vi "Amplitude and period panel.vi"() -> ()   [LabVIEW 2017]
uses:
  <vilib>/Analysis/6fits.llb/Remove Outliers (Index).vi
  control panel globals.vi
  <vilib>/Analysis/NI_AALPro.lvlib
  <vilib>/Analysis/NI_AALBase.lvlib
panel:
  in  "full x-range?":bool
  out "XY Graph":cluster{i32[], i16[]}[](graph)
  in  "discard outliers?":bool
  out "min T":dbl
  out "max T":dbl
  out "range (ms)":dbl format="%#_3f"
  out "average period (s)":dbl format="%.4f"
  out "stdev of period (ms)":dbl format="%_3f"
  out "L (m)":dbl
  in  "take snapshot":bool
  out "amplitude (mm)":sgl
  in  "clear orbit data":bool
  out "axis vs time":cluster{dbl[], dbl[]}(graph)
  out "deltaT vs. ampltidue":cluster{dbl[], dbl[]}[](graph)
  out "error out":errorcluster
  in  "log-log ?":bool
  in  "show most recent ____ seconds":dbl=5000.0
  out "period  vs time":cluster{dbl[], "dX/dt":dbl[]}(graph)
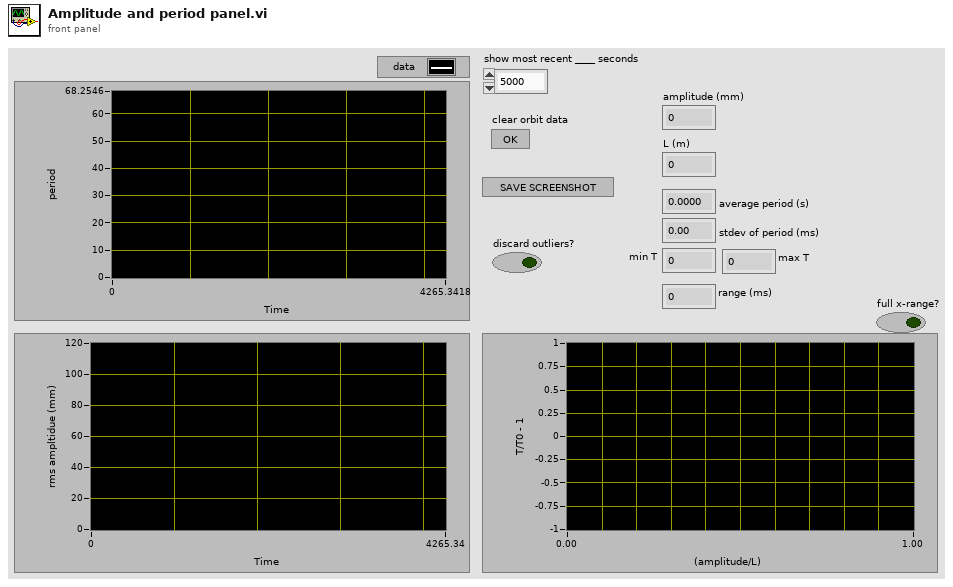
[diagram p1: front panel]
types:
  T1 = typedef "queue cluster.ctl" = cluster{"voltage":T2, "coil":T2, "mag":refnum<queue>, "accel":T2, "crossing":T2, "orbit fit":refnum<queue>, "pulse":T2, "mag0":T2, "fitLocation":refnum<queue>}
  T2 = typedef "reading queue.ctl" = refnum<queue>
  T3 = typedef "orbit parameters with crossing info.ctl" = cluster{"a":dbl, "b":dbl, "theta_axis":dbl, "dPhi":dbl, "BrV":dbl, "bob tilt":dbl, "phi0":dbl, "phi_dot":dbl, "x0":dbl, "y0":dbl, "z0":dbl, "mid crossing time":dbl, "most recent crossing number":dbl, "most recent crossing slope":dbl, "most recent crossing period":dbl}
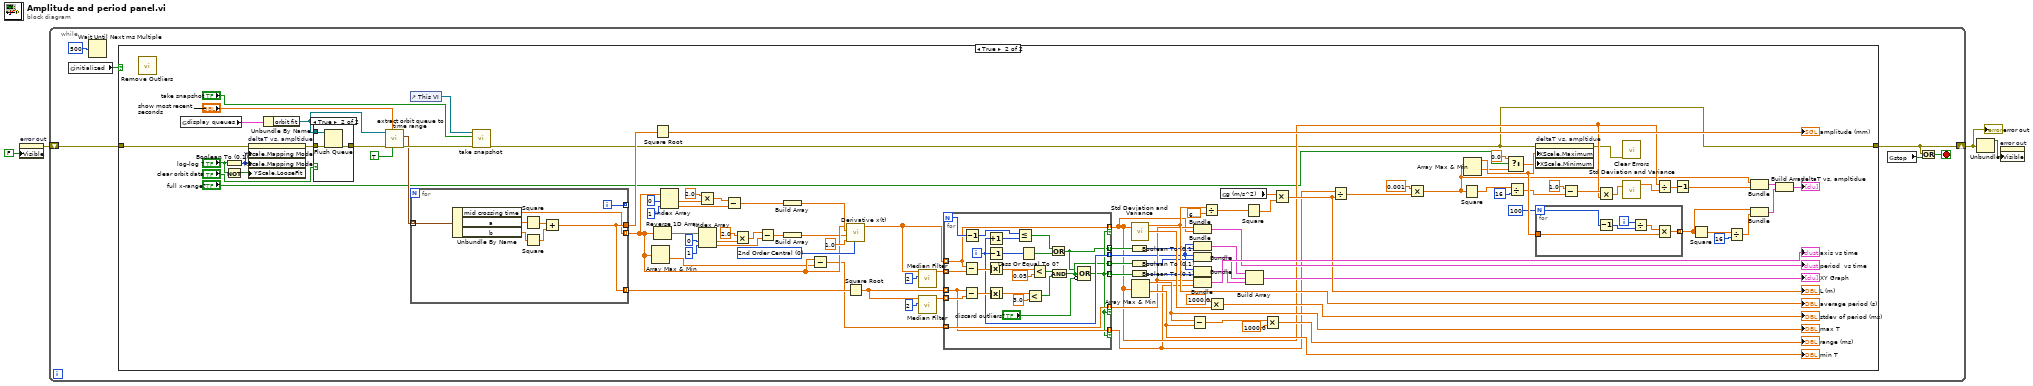
[diagram p0: block diagram]
diagram:
  n1 = property on="error out" class="Clust (strict)"("Visible"=FALSE) -> (error out=w4:errorcluster)  [unwired: 2 in, 1 out]
  n2 = while {
    shift-right: [w8] -> w2
    shift-left: w4 -> [w9]
    stop <- w7 stop-if-true
    n3 = global read "control panel globals.vi" "initialized"() -> (w10:bool)
    n4 = Wait Until Next ms Multiple(millisecond multiple=u32 500) -> ()  [unwired: 1 out]
    n5 = case shown="True" w10 {
      tunnel: [w11 w13] -> w8
      tunnel: w9 -> [w11 w113]
      frame False {
      }
      frame True {
        w96 = u16 0 items=["2nd Order Central", "4th Order Central", "Forward", "Backward"] ("method")
        n6 = call-poly <vilib>:"Remove Outliers.vi"() -> ()  [unwired: 12 in, 4 out]
        n7 = global read "control panel globals.vi" "display queues"() -> (w114:T1)
        n8 = Boolean To (0,1)(Boolean="log-log ?") -> (0, 1=w111:i16)
        n9 = Not(x="log-log ?") -> (.not. x?=w105:bool)
        n10 = property on="deltaT vs. ampltidue" class="XYGraph (strict)"(error in=w113, "YScale.Mapping Mode"=w111, "XScale.Mapping Mode"=w111, "YScale.LooseFit"=w105) -> (error out=w108:errorcluster)  [unwired: 1 in, 1 out]
        n11 = Unbundle By Name(w114) -> ("orbit fit"=w99:refnum<queue>)
        n12 = case shown="True" "clear orbit data" {
          tunnel: w108 -> [w145 w146]
          tunnel: [w145 w148] -> w107
          tunnel: w99 -> [_ w147]
          frame False {
          }
          frame True {
            n13 = Flush Queue(queue=w147, error in (no error)=w146) -> (error out=w148:errorcluster)  [unwired: 2 out]
          }
        }
        n14 = call "extract orbit queue to time range.vi"("most recent?"=TRUE, "recent interval"="show most recent ____ seconds", "error in (no error)"=w107, "orbit fit"=w99) -> ("error out"=w101:errorcluster, "extracted elements"=w48:T3[])  [unwired: 6 in]
        n15 = control-ref of="This VI"() -> (w102:refnum<vi>)
        n16 = for {
          tunnel: w48 -> [w156] mode=indexing
          tunnel: [w152] -> w104 mode=indexing
          tunnel: [w150] -> w74 mode=indexing
          tunnel: [w152] -> w103
          tunnel: [w151] -> _ mode=indexing
          i -> [w151]
          n17 = Unbundle By Name(w156) -> ("mid crossing time"=w150:dbl, "a"=w149:dbl, "b"=w155:dbl)
          n18 = Square(x=w149) -> (x^2=w153:dbl)
          n19 = Square(x=w155) -> (x^2=w154:dbl)
          n20 = Add(x=w153, y=w154) -> (x+y=w152:dbl)
        }
        n21 = call "take snapshot.vi"("error in (no error)"=w101, "take snapshot"="take snapshot", "vi ref"=w102) -> ("error out"=w13:errorcluster)  [unwired: 8 in]
        n22 = Array Max & Min(array=w74) -> (min value=w64:dbl)  [unwired: 3 out]
        n23 = Square Root(x=w103) -> (sqrt(x)=→"amplitude (mm)":dbl)
        n24 = Reverse 1D Array(array=w74) -> (reversed array=w67:dbl[])
        n25 = Index Array(array=w74, index #1=0 ("index"), index #2=1 ("index")) -> (element #1=w80:dbl, element #2=w77:dbl)
        n26 = Multiply(x=2.0, y=w80) -> (x*y=w78:dbl)
        n27 = Index Array(array=w67, index #1=0 ("index"), index #2=1 ("index")) -> (element #1=w71:dbl, element #2=w68:dbl)
        n28 = Subtract(x=w78, y=w77) -> (x-y=w76:dbl)
        n29 = Multiply(x=2.0, y=w71) -> (x*y=w69:dbl)
        n30 = Subtract(x=w69, y=w68) -> (x-y=w66:dbl)
        n31 = Build Array(w76) -> (w75:dbl[])
        n32 = Build Array(w66) -> (w65:dbl[])
        n33 = Subtract(x=w74, y=w64) -> (x-y=w42:dbl[])
        n34 = call <vilib>:"Derivative x(t).vi"("method"=w96, "dt"=1.0, "Final Condition"=w65, "Initial Condition"=w75, "X"=w74) -> ("dX/dt"=w40:dbl[])  [unwired: 5 in, 1 out]
        n35 = Square Root(x=w104) -> (sqrt(x)=w46:dbl[])
        n36 = call <vilib>:"Median Filter.vi"("left rank"=2, "X"=w40) -> ("Filtered X"=w39:dbl[])  [unwired: 8 in, 1 out]
        n37 = call <vilib>:"Median Filter.vi"("left rank"=2, "X"=w46) -> ("Filtered X"=w45:dbl[])  [unwired: 8 in, 1 out]
        n38 = for {
          N -> [w136]
          tunnel: w40 -> [w133] mode=indexing
          tunnel: w46 -> [w131] mode=indexing
          tunnel: w45 -> [w142] mode=indexing
          tunnel: w39 -> [w138] mode=indexing
          tunnel: [w133] -> w26 mode=indexing if=w123
          tunnel: [w131] -> w25 mode=indexing if=w123
          tunnel: w42 -> [w132] mode=indexing
          tunnel: [w132] -> w41 mode=indexing if=w123
          tunnel: [w124] -> w31 mode=indexing
          tunnel: [w123] -> w37 mode=indexing
          tunnel: [w122] -> w34 mode=indexing
          tunnel: [w121] -> w30 mode=indexing
          i -> [w124]
          n39 = Subtract(x=w133, y=w138) -> (x-y=w144:dbl)
          n40 = Subtract(x=w131, y=w142) -> (x-y=w141:dbl)
          n41 = Decrement(x=w136) -> (x-1=w137:i32)
          n42 = Increment(x=w124) -> (x+1=w127:i32)
          n43 = Decrement(x=w124) -> (x-1=w128:i32)
          n44 = Absolute Value(x=w144) -> (abs(x)=w143:dbl)
          n45 = Absolute Value(x=w141) -> (abs(x)=w140:dbl)
          n46 = Less Or Equal?(x=w137, y=w127) -> (x <= y?=w125:bool)
          n47 = Less Or Equal To 0?(x=w128) -> (x <= 0?=w126:bool)
          n48 = Less?(x=w140, y=3.0) -> (x < y?=w129:bool)
          n49 = Less?(x=w143, y=0.05) -> (x < y?=w135:bool)
          n50 = Or(x=w125, y=w126) -> (x .or. y?=w121:bool)
          n51 = And(x=w135, y=w129) -> (x .and. y?=w122:bool)
          n52 = Compound Arithmetic op=OR(w121, w122, invert "discard outliers?") -> (w123:bool)
        }
        n53 = Boolean To (0,1)(Boolean=w30) -> (0, 1=w29:i16[])
        n54 = Boolean To (0,1)(Boolean=w34) -> (0, 1=w33:i16[])
        n55 = Boolean To (0,1)(Boolean=w37) -> (0, 1=w36:i16[])
        n56 = call <vilib>:"Std Deviation and Variance.vi"("X"=w26) -> ("mean"=w44:dbl, "standard deviation"=w43:dbl)  [unwired: 1 in, 1 out]
        "average period (s)" <- w44
        n57 = Array Max & Min(array=w26) -> (max value=w63:dbl, min value=w56:dbl)  [unwired: 2 out]
        "max T" <- w63
        "min T" <- w56
        n58 = Subtract(x=w63, y=w56) -> (x-y=w62:dbl)
        n59 = Bundle(w41, w26) -> (→"period  vs time":cluster{dbl[], dbl[]})  [unwired: 1 in]
        n60 = Bundle(w31, w29) -> (w27:cluster{i32[], i16[]})  [unwired: 1 in]
        n61 = Bundle(w31, w33) -> (w32:cluster{i32[], i16[]})  [unwired: 1 in]
        n62 = Bundle(w31, w36) -> (w35:cluster{i32[], i16[]})  [unwired: 1 in]
        n63 = Bundle(w41, w25) -> (→"axis vs time":cluster{dbl[], dbl[]})  [unwired: 1 in]
        n64 = Divide(x=w44, y=6.283185307179586) -> (x/y=w90:dbl)
        n65 = Multiply(x=1000.0, y=w43) -> (x*y=→"stdev of period (ms)":dbl)
        n66 = global read "control panel globals.vi" "g (m/s^2)"() -> (w92:dbl)
        n67 = Square(x=w90) -> (x^2=w89:dbl)
        n68 = Build Array(w27, w32, w35) -> (→"XY Graph":cluster{i32[], i16[]}[])
        n69 = Multiply(x=w62, y=1000.0) -> (x*y=→"range (ms)":dbl)
        n70 = Multiply(x=w92, y=w89) -> (x*y=w57:dbl)
        "L (m)" <- w57
        n71 = Divide(x=w25, y=w57) -> (x/y=w88:dbl[])
        n72 = Multiply(x=0.001, y=w88) -> (x*y=w19:dbl[])
        n73 = Square(x=w19) -> (x^2=w21:dbl[])
        n74 = Array Max & Min(array=w19) -> (max value=w24:dbl, min value=w16:dbl)  [unwired: 2 out]
        n75 = Select(t=0.0, s="full x-range?", f=w16) -> (s? t:f=w14:dbl)
        n76 = Divide(x=w21, y=16) -> (x/y=w18:dbl[])
        n77 = property on="deltaT vs. ampltidue" class="XYGraph (strict)"(error in=w13, "XScale.Maximum"=w24, "XScale.Minimum"=w14) -> (error out=w12:errorcluster)  [unwired: 1 in, 1 out]
        n78 = for {
          N: 100 -> [w119]
          tunnel: w24 -> [w117]
          tunnel: [w115] -> w22 mode=indexing
          i -> [w120]
          n79 = Decrement(x=w119) -> (x-1=w116:i32)
          n80 = Divide(x=w120, y=w116) -> (x/y=w118:dbl)
          n81 = Multiply(x=w118, y=w117) -> (x*y=w115:dbl)
        }
        n82 = Subtract(x=1.0, y=w18) -> (x-y=w51:dbl[])
        n83 = Multiply(x=w51, y=w26) -> (x*y=w50:dbl[])
        n84 = call <vilib>:"Clear Errors.vi"("error in (no error)"=w12) -> ()  [unwired: 5 in, 2 out]
        n85 = call <vilib>:"Std Deviation and Variance.vi"("X"=w50) -> ("mean"=w49:dbl)  [unwired: 1 in, 2 out]
        n86 = Divide(x=w26, y=w49) -> (x/y=w94:dbl[])
        n87 = Decrement(x=w94) -> (x-1=w93:dbl[])
        n88 = Square(x=w22) -> (x^2=w61:dbl[])
        n89 = Divide(x=w61, y=16) -> (x/y=w53:dbl[])
        n90 = Bundle(w19, w93) -> (w87:cluster{dbl[], dbl[]})  [unwired: 1 in]
        n91 = Bundle(w22, w53) -> (w58:cluster{dbl[], dbl[]})  [unwired: 1 in]
        n92 = Build Array(w87, w58) -> (→"deltaT vs. ampltidue":cluster{dbl[], dbl[]}[])
      }
    }
    n93 = global read "control panel globals.vi" "stop"() -> (w6:bool)
    n94 = Or(x=w8, y=w6) -> (x .or. y?=w7:bool)
  }
  "error out" <- w2
  n95 = Unbundle(w2) -> ("status"=w1:bool)  [unwired: 2 out]
  n96 = property on="error out" class="Clust (strict)"("Visible"=w1) -> ()  [unwired: 2 in, 2 out]
